vi "Update Mouse Up.vi"(8 "error in (no error)":errorcluster, 10 "Mouse Up":T1, 11 "Map Model in":refnum<class "Map Model.lvclass">) -> (0 "error out":errorcluster, 3 "Map Model out":refnum<class "Map Model.lvclass">)   [LabVIEW 2020, in "Map Model.lvlib" / "Map Model.lvclass"]
uses:
  Map Model.lvclass
  <vilib>/Utility/miscctls.llb/LVPoint32TypeDef.ctl
  Map Model.lvclass/Map Model.ctl
  Tools/Tool/Tool.lvclass/Tool.ctl
  Tools/Tool/Tool.lvclass
panel:
  # "NOTICE -- YOU MUST LEAVE THIS NOTICE IN PLACE.\n\nCopyright (c) 2017, LIANG LIU Shawn.Liu.cn@gmail.com\nAll rights reserved.\n\nRedistribution and use in source and binary forms, with or without modification, are permitted provided that the following conditions are met:\n-Redistributions of source code must retain the above copyright notice, this list of conditions and the following disclaimer.\n-Redistributions in binary form must reproduce the above copyright notice, this list of conditions and the following disclaimer in the documentation and/or other materials provided with the distribution.\n-Neither the name of the eLp nor the names of its contributors may be used to endorse or promote products derived from this software without specific prior written permission.\n\nTHIS SOFTWARE IS PROVIDED BY THE COPYRIGHT HOLDERS AND CONTRIBUTORS \"AS IS\" AND ANY EXPRESS OR IMPLIED WARRANTIES, INCLUDING, BUT NOT LIMITED TO, THE IMPLIED WARRANTIES OF MERCHANTABILITY AND FITNESS FOR A PARTICULAR PURPOSE ARE DISCLAIMED. IN NO EVENT SHALL THE COPYRIGHT HOLDER OR CONTRIBUTORS BE LIABLE FOR ANY DIRECT, INDIRECT, INCIDENTAL, SPECIAL, EXEMPLARY, OR CONSEQUENTIAL DAMAGES (INCLUDING, BUT NOT LIMITED TO, PROCUREMENT OF SUBSTITUTE GOODS OR SERVICES; LOSS OF USE, DATA, OR PROFITS; OR BUSINESS INTERRUPTION) HOWEVER CAUSED AND ON ANY THEORY OF LIABILITY, WHETHER IN CONTRACT, STRICT LIABILITY, OR TORT (INCLUDING NEGLIGENCE OR OTHERWISE) ARISING IN ANY WAY OUT OF THE USE OF THIS SOFTWARE, EVEN IF ADVISED OF THE POSSIBILITY OF SUCH DAMAGE."
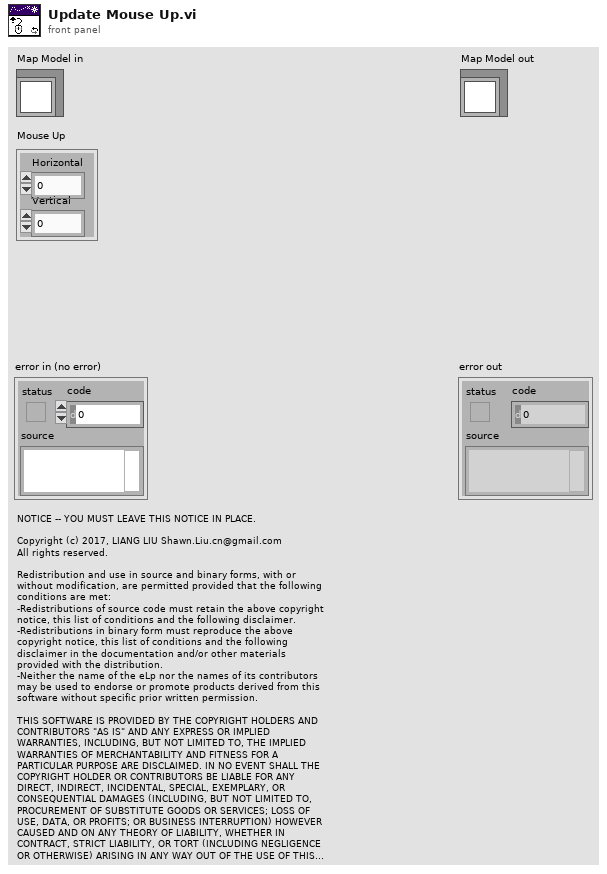
[diagram p1: front panel]
types:
  T1 = typedef "LVPoint32TypeDef.ctl" = cluster{"Horizontal":i32, "Vertical":i32}
  T2 = enum8{"Enabled", "Disabled", "Disabled and Grayed Out"}
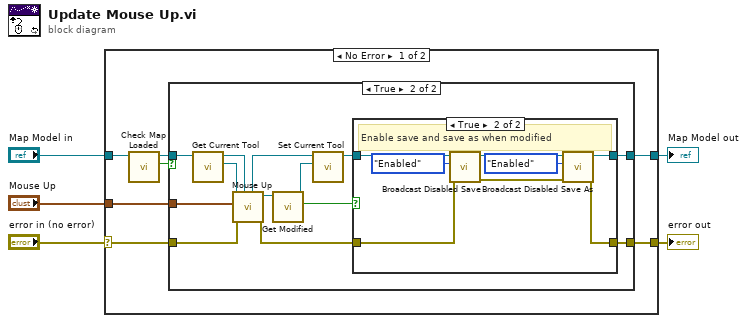
[diagram p0: block diagram]
diagram:
  n1 = case shown="No Error" "error in (no error)" {
    selector: "error in (no error)" -> [w8 w39]
    tunnel: "Map Model in" -> [w12 w38]
    tunnel: [w11 w38] -> w4
    tunnel: [w10 w39] -> w3
    tunnel: "Mouse Up" -> [w9 _]
    frame No Error {
      n2 = call "Check Map Loaded.vi"("Map Model in"=w12) -> ("Loaded"=w6:bool, "Map Model out"=w7:refnum<class "Map Model.lvclass">)  [unwired: 9 in]
      n3 = case shown="True" w6 {
        tunnel: [w14 w20] -> w11
        tunnel: w9 -> [_ w27]
        tunnel: [w13 w19] -> w10
        tunnel: w7 -> [w14 w24]
        tunnel: w8 -> [w13 w22]
        frame False {
        }
        frame True {
          n4 = call "Get Current Tool.vi"("Map Model in"=w24) -> ("Current Tool"=w23:refnum<class "Tool.lvclass">, "Map Model out"=w26:refnum<class "Map Model.lvclass">)  [unwired: 9 in]
          n5 = call-dynamic "Mouse Up.vi"("Map Model in"=w26, "error in (no error)"=w22, "Position"=w27, "Tool in"=w23) -> ("error out"=w15:errorcluster, "Tool out"=w17:refnum<class "Tool.lvclass">, "Map Model out"=w25:refnum<class "Map Model.lvclass">)  [unwired: 5 in]
          n6 = call "Get Modified.vi"("Tool in"=w17) -> ("Modified"=w16:bool, "Tool out"=w18:refnum<class "Tool.lvclass">)  [unwired: 9 in]
          n7 = call "Set Current Tool.vi"("Current Tool"=w18, "Map Model in"=w25) -> ("Map Model out"=w21:refnum<class "Map Model.lvclass">)  [unwired: 9 in]
          n8 = case shown="True" w16 {
            tunnel: w21 -> [w29 w35]
            tunnel: [w29 w34] -> w20
            tunnel: [w28 w33] -> w19
            tunnel: w15 -> [w28 w30]
            frame False {
            }
            frame True {
              # "Enable save and save as when modified"
              n9 = call "Broadcast Disabled Save.vi"("error in (no error)"=w30, "Disabled Save"=T2."Enabled", "Map Model in"=w35) -> ("error out"=w36:errorcluster, "Map Model out"=w37:refnum<class "Map Model.lvclass">)  [unwired: 7 in]
              n10 = call "Broadcast Disabled Save As.vi"("error in (no error)"=w36, "Disabled Save As"=T2."Enabled", "Map Model in"=w37) -> ("error out"=w33:errorcluster, "Map Model out"=w34:refnum<class "Map Model.lvclass">)  [unwired: 7 in]
            }
          }
        }
      }
    }
    frame Error {
    }
  }
  "error out" <- w3
  "Map Model out" <- w4
